vi "FloorTest.vi"() -> ()   [LabVIEW 2013]
panel:
  in  "Tab Control":enum32{"All DBL", "From Lua"}(tab)
  out "delays":dbl[](array[numeric])
  out "# steps DBL\n(round -> -inf)":dbl[](array[numeric]) format="%#_15g"
  out "# steps I32\n(round -> -inf) 2":i32[](array[numeric])
  out "# steps 2 DBL\n(form node: floor)":dbl[](array[numeric])
  out "# steps 2 DBL\n(form node: floor) 2":i32[](array[numeric])
  out "delays (str, %p)":string[](array[string])
  out "delays (str, %15p) 2":string[](array[string])
  in  "step":dbl
  in  "num pnts":dbl
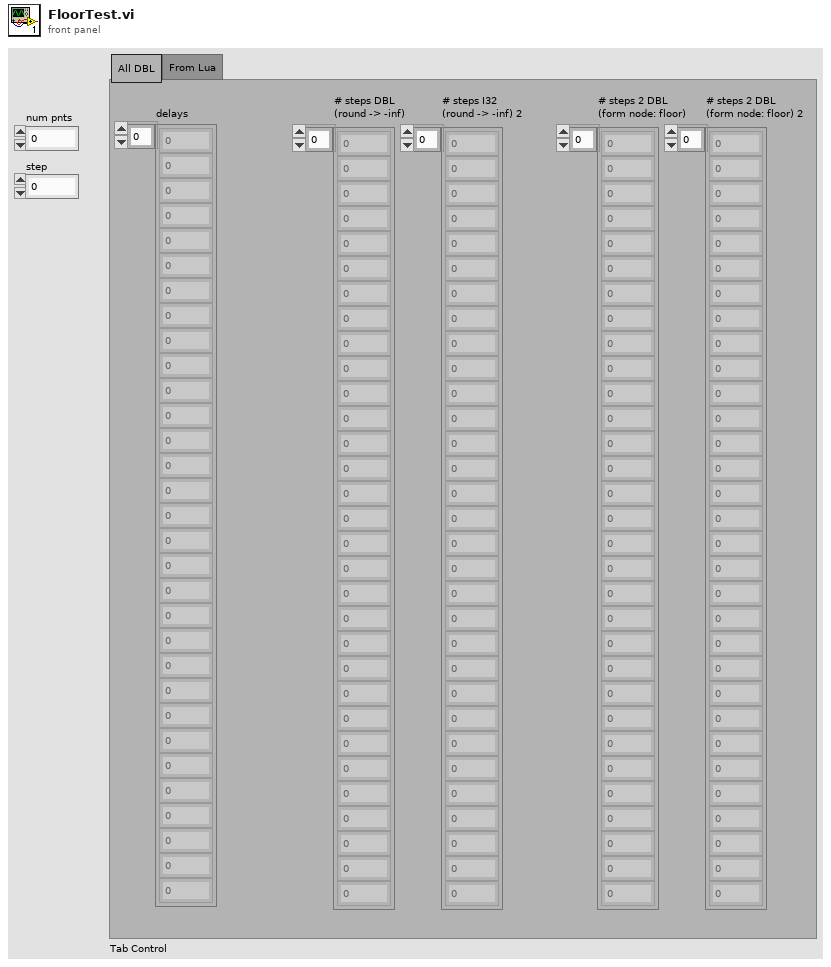
[diagram p1: front panel]
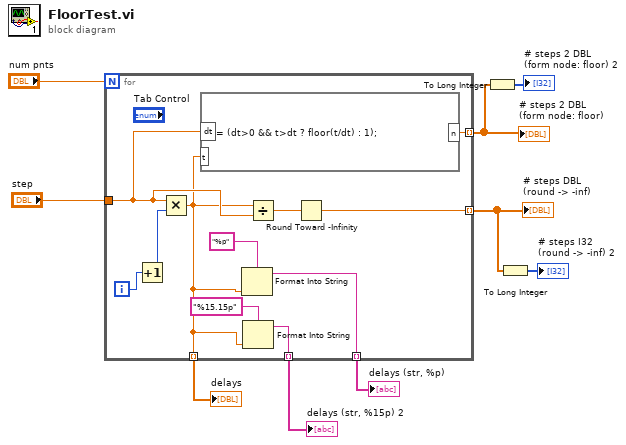
[diagram p0: block diagram]
diagram:
  n1 = for {
    N: "num pnts" -> [_]
    tunnel: "step" -> [w15]
    tunnel: [w11] -> w3 mode=indexing
    tunnel: [w17] -> w6 mode=indexing
    tunnel: [w16] -> w4 mode=indexing
    tunnel: [w14] -> w2 mode=indexing
    tunnel: [w10] -> w1 mode=indexing
    i -> [w20]
    n2 = Increment(x=w20) -> (x+1=w19:i32)
    n3 = Multiply(x=w15, y=w19) -> (x*y=w11:dbl)
    n4 = formula code="n= (dt>0 && t>dt ? floor(t/dt) : 1);"("dt"=w15, "t"=w11) -> ("n"=w16:dbl)
    n5 = Format Into String(format string="%p", w11) -> (resulting string=w14:string)  [unwired: 2 in, 1 out]
    n6 = Format Into String(format string="%15.15p", w11) -> (resulting string=w10:string)  [unwired: 2 in, 1 out]
    n7 = Divide(x=w11, y=w15) -> (x/y=w18:dbl)
    n8 = Round Toward -Infinity(1:w18) -> (0:w17:dbl)
  }
  "delays" <- w3
  "# steps DBL\n(round -> -inf)" <- w6
  "# steps 2 DBL\n(form node: floor)" <- w4
  "delays (str, %p)" <- w2
  "delays (str, %15p) 2" <- w1
  n9 = To Long Integer(number=w4) -> (32bit integer=→"# steps 2 DBL\n(form node: floor) 2":i32[])
  n10 = To Long Integer(number=w6) -> (32bit integer=→"# steps I32\n(round -> -inf) 2":i32[])
